vi "Create.vi"(8 "error in (no error)":errorcluster, 9 "Col":u64, 10 "Row":u64) -> (0 "error out":errorcluster, 3 "Galaxy":refnum<class "Galaxy.lvclass">)   [LabVIEW 2020, in "Galaxy.lvclass"]
uses:
  Galaxy.lvclass
  Galaxy.lvclass/Galaxy.ctl
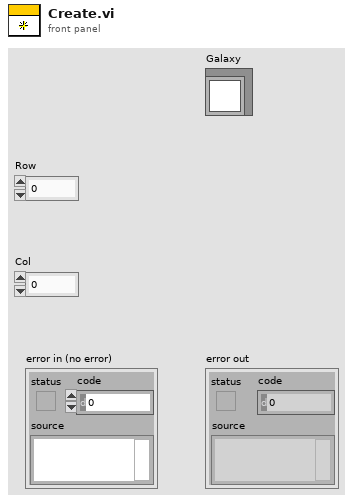
[diagram p1: front panel]
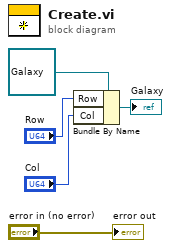
[diagram p0: block diagram]
diagram:
  n1 = Bundle By Name(cluster=refnum<class "Galaxy.lvclass"> refnum ("Galaxy"), "Row"="Row", "Col"="Col") -> (→"Galaxy":refnum<class "Galaxy.lvclass">)
  "error out" <- "error in (no error)"
